vi "病人基本信息读取.vi"() -> ()   [LabVIEW 2018]
uses:
  <vilib>/Utility/file.llb/Read Delimited Spreadsheet (string).vi
panel:
  out "all rows":string[][](array[string]) caption="所有行"
  in  "按钮 3":bool
  in  "按钮 2":bool
  in  "按钮":bool
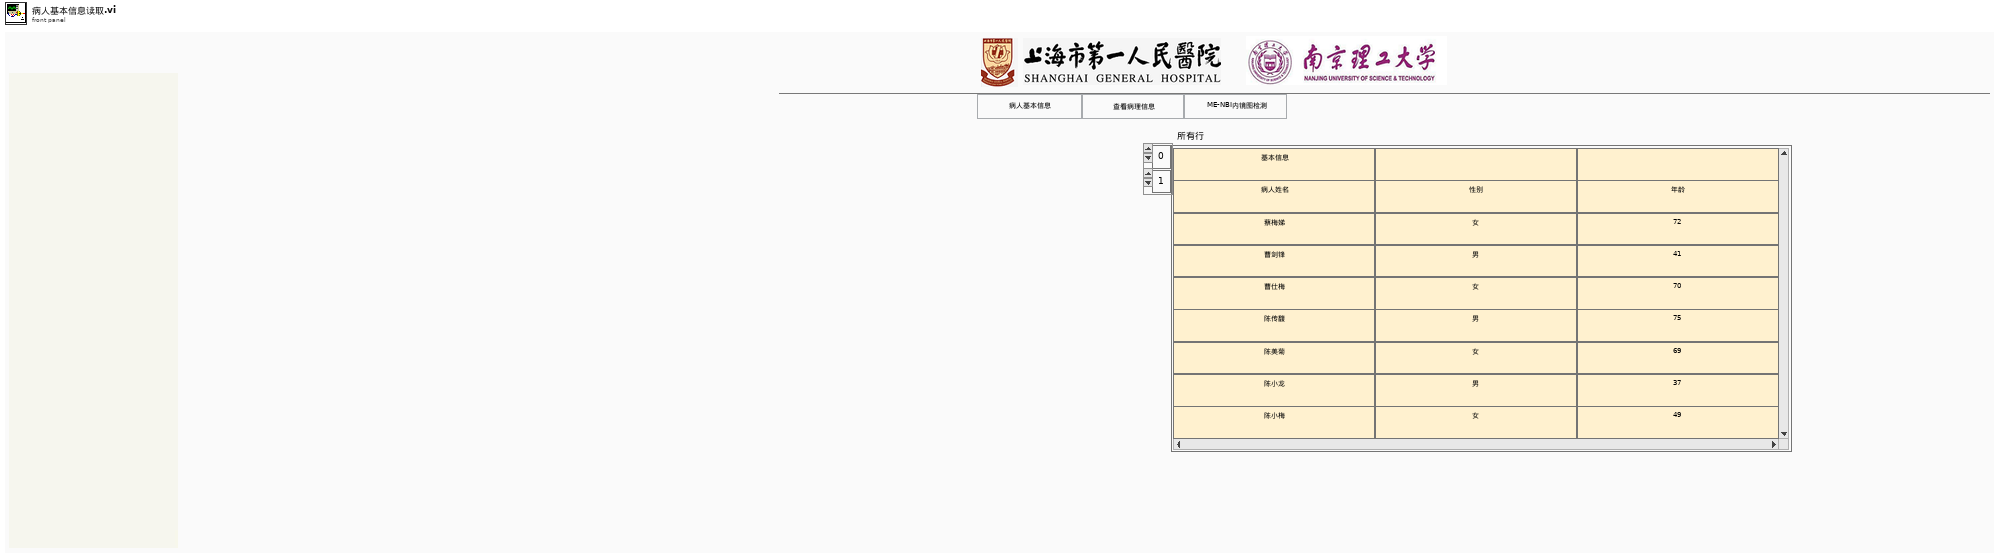
[diagram p1: front panel]
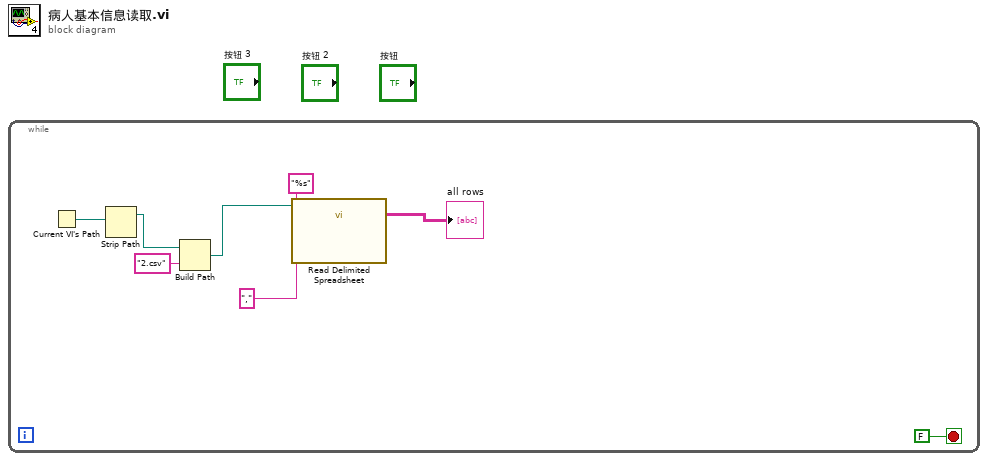
[diagram p0: block diagram]
diagram:
  n1 = while {
    stop <- FALSE stop-if-true
    n2 = Current VI's Path() -> (path=w8:path)
    n3 = Strip Path(path=w8) -> (stripped path=w7:path)  [unwired: 1 out]
    n4 = Build Path(base path=w7, name or relative path="2.csv" ("名称或相对路径")) -> (appended path=w5:path)
    n5 = call-poly <vilib>:"Read Delimited Spreadsheet.vi"("file path (dialog if empty)"=w5, "format (%s)"="%s", "delimiter (\\t)"="," ("delimiter (\\t)")) -> ("all rows"=→"all rows":string[][])  [unwired: 7 in, 5 out]
  }
